vi "Get_initialize_Config.vi"() -> (3 "Local Database":bool)   [LabVIEW 2011]
uses:
  <vilib>/Utility/file.llb/Read From Spreadsheet File (string).vi
panel:
  out "all rows":string[][](array[string]) caption="所有行"
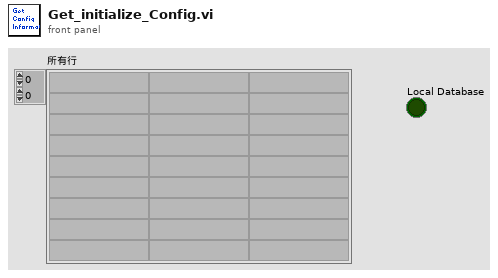
[diagram p1: front panel]
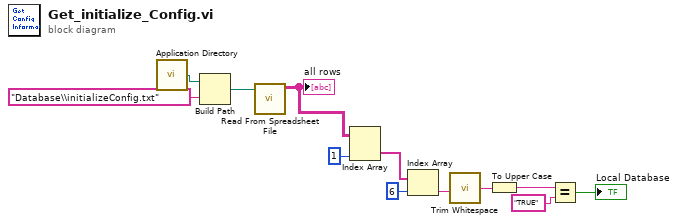
[diagram p0: block diagram]
diagram:
  n1 = call <vilib>:"Application Directory.vi"() -> ("Application Directory"=w12:path)
  n2 = Build Path(base path=w12, name or relative path="Database\\initializeConfig.txt" ("名称或相对路径")) -> (appended path=w10:path)
  n3 = call-poly <vilib>:"Read From Spreadsheet File.vi"("file path (dialog if empty)"=w10) -> ("all rows"=w9:string[][])  [unwired: 6 in, 4 out]
  "all rows" <- w9
  n4 = Index Array(array=w9, index (col)=1 ("禁用的索引 (列)")) -> (element=w7:string[])  [unwired: 1 in]
  n5 = Index Array(array=w7, index=6 ("索引")) -> (element=w3:string)
  n6 = call <vilib>:"Trim Whitespace.vi"("string"=w3) -> ("trimmed string"=w2:string)  [unwired: 1 in]
  n7 = To Upper Case(1:w2) -> (0:w1:string)
  n8 = Equal?(x=w1, y="TRUE") -> (x = y?=→"Local Database":bool)
